vi "Roi_aus_position.vi"() -> ()   [LabVIEW 2014]
uses:
  <vilib>/vision/Image Controls.llb/IMAQ Image.ctl
  <vilib>/userdefined/High Color/IMAQdx.ctl
  <vilib>/vision/driver/NI_Vision_Acquisition_Software.lvlib
  <vilib>/vision/NI_Vision_Development_Module.lvlib
panel:
  in  "Advanced Options":cluster{"Item":u16, "Value":dbl}[](array[cluster]) {"Item" items=["LD Sampling - Search Strategy Support"=0, "LD Sampling - Initial Step Size"=1, "LD Sampling - Initial Sample Size"=2, "LD Sampling - Initial Sample Size Factor"=3, "LD Sampling - Initial Angular Accuracy"=4, "LD Sampling - Final Sample Size"=5, "LD Sampling - Final Sample Size Factor"=6, "LD Sampling - Final Angular Accuracy"=7, "LD Sampling - Subpixel Sample Size"=8, "LD Sampling - Subpixel Sample Size Factor"=9, "LD Sampling - Match Offset X Position"=10, "LD Sampling - Match Offset Y Position"=11, "LD Sampling - Match Offset Angle"=12, "-"=13, "Pyramid - Subpixel Sample Size"=100, "Pyramid - Subpixel Sample Size Factor"=101, "Pyramid - Match Offset X Position"=102, "Pyramid - Match Offset Y Position"=103, "Pyramid - Match Offset Angle"=104, "Pyramid - Max Pyramid Level To Store Data"=105]}
  in  "Image":T1
  out "Template":T1(plugin-control)
  in  "Replace Value":sgl=1.0 format="%.2f"
  in  "Keep/Replace Value (Replace) 2":bool=TRUE
  in  "Range":cluster{"Lower value":sgl, "Upper value":sgl}={"Lower value"=128.0, "Upper value"=255.0} {"Upper value" format="%.2f"; "Lower value" format="%.2f"}
  out "Threshold Image 2":T1(plugin-control)
  in  "stop":bool
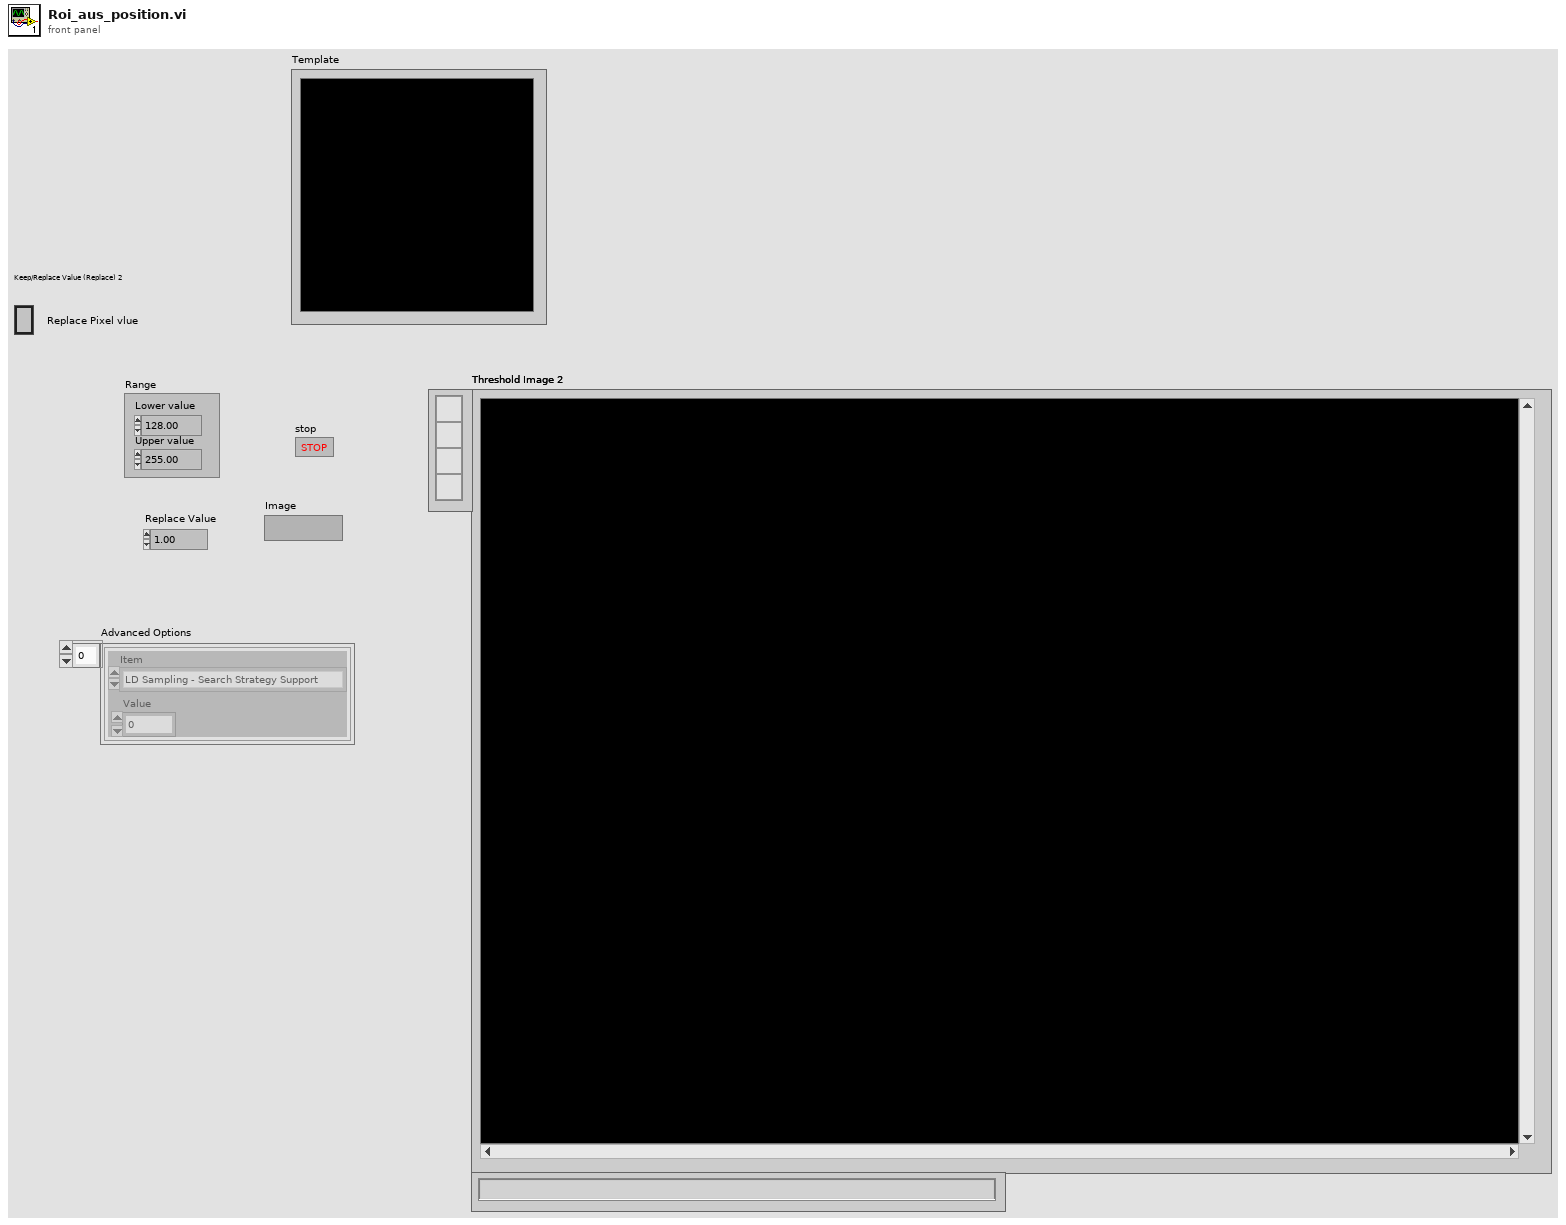
[diagram p1: front panel]
types:
  T1 = typedef "IMAQ Image.ctl" = refnum<image>
  T2 = typedef "Image Type" = u32
  T3 = typedef "IMAQdx.ctl" = refnum<k21>
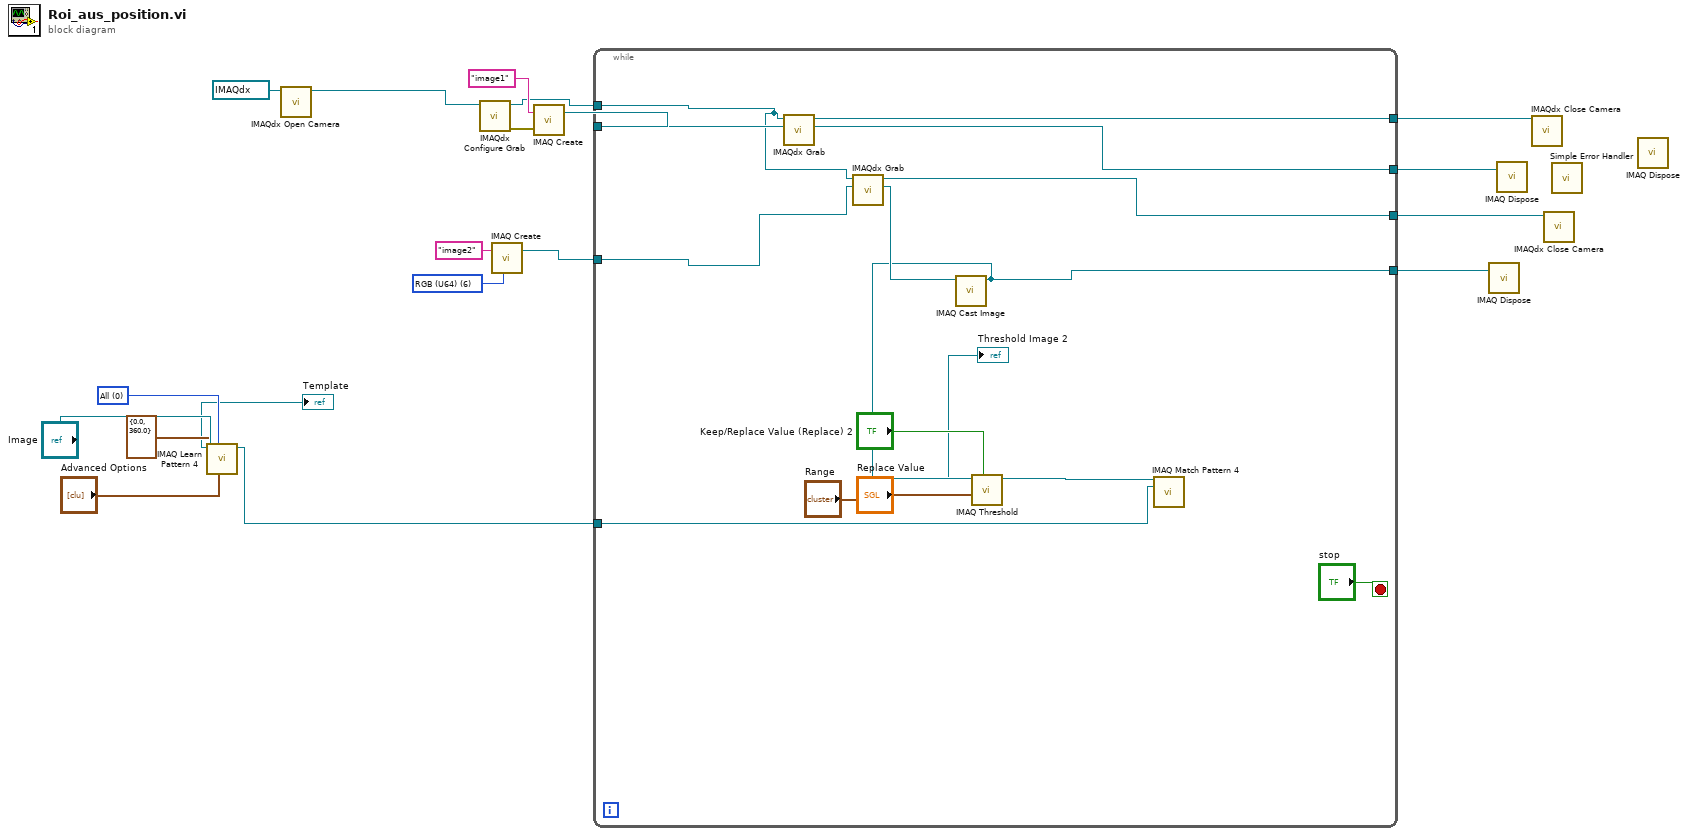
[diagram p0: block diagram]
diagram:
  w5 = 0 items=["All", "Low Discrepancy Sampling", "Grayscale Value Pyramid", "Gradients Pyramid"] ("Algorithm")
  w13 = T2 6 items=["Grayscale (U8)", "Grayscale (I16)", "Grayscale (SGL)", "Complex (CSG)", "RGB (U32)", "HSL (U32)", "RGB (U64)", "Grayscale (U16)"] ("Image Type")
  n1 = call "IMAQ Learn Pattern 4"("Advanced Options"="Advanced Options", "Algorithm"=w5, "Angle Range"=cluster{"Start Angle":sgl, "End Angle":sgl} {"Start Angle"=0.0, "End Angle"=360.0}, "Image"="Image") -> ("Template Image Out"=w1:T1)  [unwired: 5 in, 2 out]
  "Template" <- w1
  n2 = call <vilib>:"IMAQdx Open Camera.vi"("Session In"=T3 "cam0") -> ("Session Out"=w15:T3)  [unwired: 9 in, 1 out]
  n3 = call <vilib>:"IMAQdx Configure Grab.vi"("Session In"=w15) -> ("error out"=w17:errorcluster, "Session Out"=w11:T3)  [unwired: 9 in]
  n4 = call "IMAQ Create"("Image Name"="image2", "Image Type"=w13) -> ("New Image"=w12:T1)  [unwired: 3 in, 1 out]
  n5 = call "IMAQ Create"("Image Name"="image1", "error in (no error)"=w17) -> ("New Image"=w10:T1)  [unwired: 3 in, 1 out]
  n6 = while {
    tunnel: w12 -> [w28]
    tunnel: w11 -> [w29]
    tunnel: w10 -> [w30]
    tunnel: [w27] -> w9
    tunnel: [w21] -> w8
    tunnel: [w26] -> w7
    tunnel: [w22] -> w6
    tunnel: w1 -> [w19]
    stop <- "stop" stop-if-true
    n7 = call <vilib>:"IMAQdx Grab.vi"("Image In"=w30, "Session In"=w29) -> ("Image Out"=w21:T1, "Session Out"=w27:T3)  [unwired: 6 in, 2 out]
    n8 = call <vilib>:"IMAQdx Grab.vi"("Image In"=w28, "Session In"=w29) -> ("Image Out"=w31:T1, "Session Out"=w26:T3)  [unwired: 6 in, 2 out]
    n9 = call "IMAQ Cast Image"("Image Src"=w31) -> ("Image Dst Out"=w22:T1)  [unwired: 9 in, 1 out]
    n10 = call "IMAQ Threshold"("Replace Value"="Replace Value", "Keep/Replace Value (Replace)"="Keep/Replace Value (Replace) 2", "Range"="Range", "Image Src"=w22) -> ("Image Dst Out"=w20:T1)  [unwired: 6 in, 1 out]
    "Threshold Image 2" <- w20
    n11 = call "IMAQ Match Pattern 4"("Image"=w20, "Template Image"=w19) -> ()  [unwired: 9 in, 5 out]
  }
  n12 = call "IMAQ Dispose"("Image"=w6) -> ()  [unwired: 5 in, 1 out]
  n13 = call "IMAQ Dispose"("Image"=w8) -> ()  [unwired: 5 in, 1 out]
  n14 = call <vilib>:"IMAQdx Close Camera.vi"("Session In"=w9) -> ()  [unwired: 10 in, 1 out]
  n15 = call <vilib>:"IMAQdx Close Camera.vi"("Session In"=w7) -> ()  [unwired: 10 in, 1 out]
  n16 = call <vilib>:"Simple Error Handler.vi"() -> ()  [unwired: 5 in, 5 out]
  n17 = call "IMAQ Dispose"() -> ()  [unwired: 6 in, 1 out]
